vi "DSF.Engine.Plugin.Tx.vi"(8 "error in (no error)":errorcluster, 11 "Plugin in":refnum<class "DSF.Engine.Plugin.lvclass">) -> (0 "error out":errorcluster, 3 "Plugin out":refnum<class "DSF.Engine.Plugin.lvclass">)   [LabVIEW 2017, in "DSF.Engine.lvlib" / "DSF.Engine.Plugin.lvclass"]
uses:
  DSF.Engine.Plugin.lvclass
  DSF.Engine.Plugin.lvclass/DSF.Engine.Plugin.ctl
  Timing/DSF.Engine.Timing.lvclass/DSF.Engine.Timing.ctl
  Transfer/DSF.Engine.Transfer Group.lvclass
  Timing/DSF.Engine.Timing.lvclass
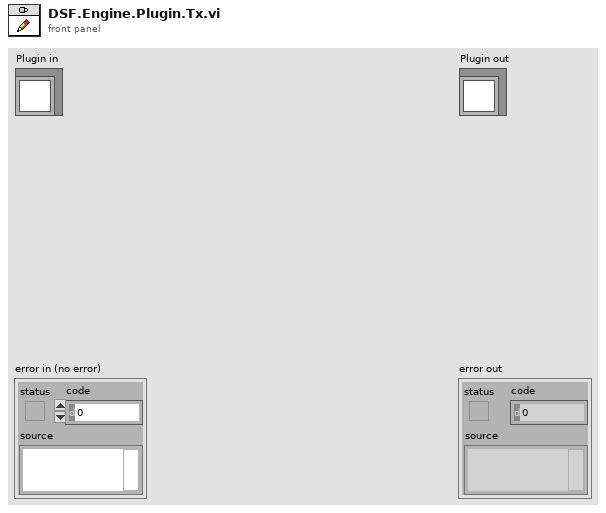
[diagram p1: front panel]
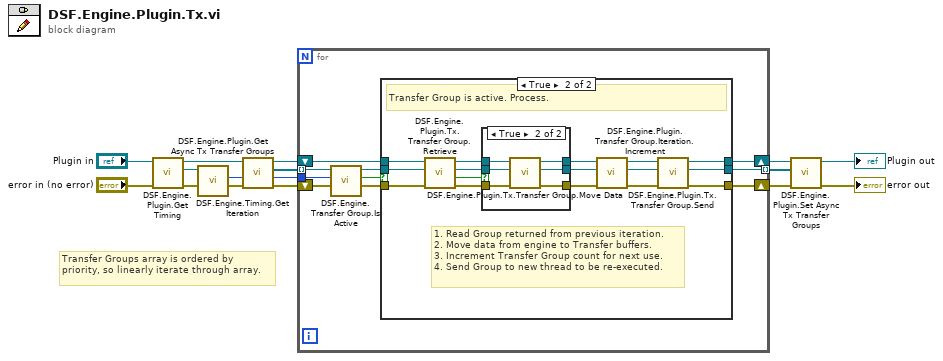
[diagram p0: block diagram]
diagram:
  # "Transfer Groups array is ordered by priority, so linearly iterate through array."
  n1 = call "DSF.Engine.Plugin.Get Timing.vi"("Plugin in"="Plugin in") -> ("Timing"=w8:refnum<class "DSF.Engine.Timing.lvclass">, "Plugin out"=w9:refnum<class "DSF.Engine.Plugin.lvclass">)  [unwired: 9 in]
  n2 = call "DSF.Engine.Timing.Get Iteration.vi"("Timing in"=w8) -> ("Iteration"=w7:u64)  [unwired: 9 in, 1 out]
  n3 = call "DSF.Engine.Plugin.Get Async Tx Transfer Groups.vi"("Plugin in"=w9) -> ("Tx Transfer Groups"=w11:refnum<class "DSF.Engine.Transfer Group.lvclass">[], "Plugin out"=w10:refnum<class "DSF.Engine.Plugin.lvclass">)  [unwired: 9 in]
  n4 = for {
    tunnel: w11 -> [w20] mode=indexing
    shift-right: [w13] -> w6
    shift-left: w10 -> [w14]
    tunnel: w7 -> [w19]
    shift-right: [w18] -> w1
    shift-left: "error in (no error)" -> [w17]
    tunnel: [w12] -> w5 mode=indexing
    n5 = call "DSF.Engine.Transfer Group.Is Active.vi"("cycle count"=w19, "Transfer Group in"=w20) -> ("active this cycle?"=w16:bool, "Transfer Group out"=w15:refnum<class "DSF.Engine.Transfer Group.lvclass">)  [unwired: 8 in]
    n6 = case shown="True" w16 {
      tunnel: [w23 w38] -> w18
      tunnel: w17 -> [w23 w36]
      tunnel: w15 -> [w21 w35]
      tunnel: w14 -> [w22 w37]
      tunnel: [w22 w39] -> w13
      tunnel: [w21 w31] -> w12
      frame False {
        # "Transfer Group is not active. Skip."
      }
      frame True {
        # "1. Read Group returned from previous iteration.\n2. Move data from engine to Transfer buffers.\n3. Increment Transfer Group count for next use.\n4. Send Group to new thread to be re-executed."
        # "Transfer Group is active. Process."
        n7 = call "DSF.Engine.Plugin.Tx.Transfer Group.Retrieve.vi"("error in (no error)"=w36, "Transfer Group in"=w35, "Plugin in"=w37) -> ("error out"=w24:errorcluster, "move data?"=w25:bool, "Transfer Group out"=w29:refnum<class "DSF.Engine.Transfer Group.lvclass">, "Plugin out"=w30:refnum<class "DSF.Engine.Plugin.lvclass">)  [unwired: 5 in]
        n8 = case shown="True" w25 {
          tunnel: w30 -> [w41 w48]
          tunnel: w29 -> [w42 w47]
          tunnel: [w41 w46] -> w28
          tunnel: [w42 w45] -> w27
          tunnel: [w40 w44] -> w26
          tunnel: w24 -> [w40 w43]
          frame False {
          }
          frame True {
            n9 = call "DSF.Engine.Plugin.Tx.Transfer Group.Move Data.vi"("error in (no error)"=w43, "Transfer Group in"=w47, "Plugin in"=w48) -> ("error out"=w44:errorcluster, "Transfer Group out"=w45:refnum<class "DSF.Engine.Transfer Group.lvclass">, "Plugin out"=w46:refnum<class "DSF.Engine.Plugin.lvclass">)  [unwired: 6 in]
          }
        }
        n10 = call "DSF.Engine.Plugin.Transfer Group.Iteration.Increment.vi"("error in (no error)"=w26, "Transfer Group in"=w27, "Plugin in"=w28) -> ("error out"=w33:errorcluster, "Transfer Group out"=w32:refnum<class "DSF.Engine.Transfer Group.lvclass">, "Plugin out"=w34:refnum<class "DSF.Engine.Plugin.lvclass">)  [unwired: 6 in]
        n11 = call "DSF.Engine.Plugin.Tx.Transfer Group.Send.vi"("error in (no error)"=w33, "Transfer Group in"=w32, "Plugin in"=w34) -> ("error out"=w38:errorcluster, "Transfer Group out"=w31:refnum<class "DSF.Engine.Transfer Group.lvclass">, "Plugin out"=w39:refnum<class "DSF.Engine.Plugin.lvclass">)  [unwired: 6 in]
      }
    }
  }
  "error out" <- w1
  n12 = call "DSF.Engine.Plugin.Set Async Tx Transfer Groups.vi"("Tx Transfer Groups"=w5, "Plugin in"=w6) -> ("Plugin out"=→"Plugin out":refnum<class "DSF.Engine.Plugin.lvclass">)  [unwired: 9 in]
